vi "DecreaseParameterBounds.vi"(8 "delta":dbl=1.0, 10 "Best Fits":dbl[](array[numeric]), 11 "parameter bounds in":T1={"parameter minimum"=[1.0, 0.0, 0.0, 1.0, 1.0, -720.0, 0.0], "parameter maximum"=[255.0, 640.0, 480.0, 80.0, 80.0, 720.0, 128.0]}) -> (3 "parameter bounds out":T1={"parameter minimum"=[1.0, 0.0, 0.0, 1.0, 1.0, -720.0, 0.0], "parameter maximum"=[255.0, 640.0, 480.0, 80.0, 80.0, 720.0, 128.0]})   [LabVIEW 2015]
panel:
  in  "Amplitude min":dbl=1.0
  # "(0) Amplitude\n(1) X-Pos\n(2) Y-Pos\n(3) width A\n(4) Width B\n(5) angle (DEG)\n(6) Offset"
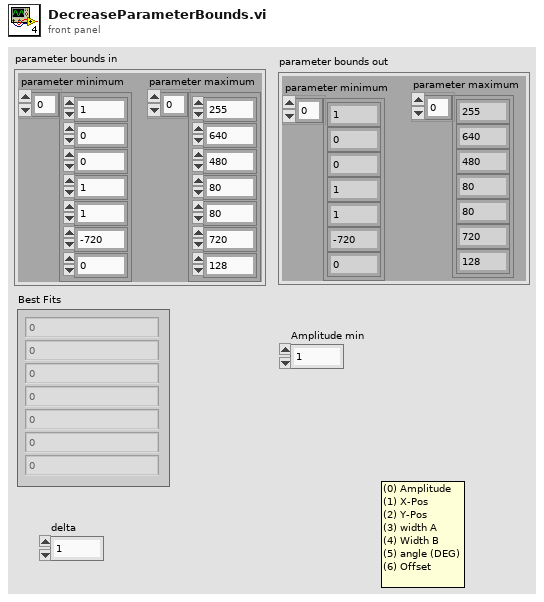
[diagram p1: front panel]
types:
  T1 = cluster{"parameter minimum":dbl[], "parameter maximum":dbl[]}
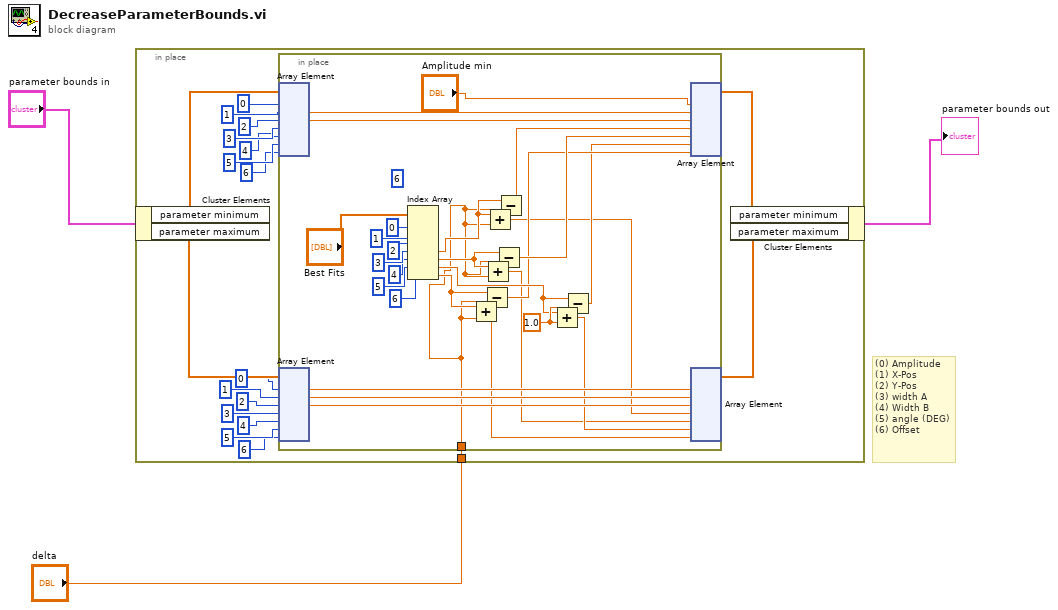
[diagram p0: block diagram]
diagram:
  # "(0) Amplitude\n(1) X-Pos\n(2) Y-Pos\n(3) width A\n(4) Width B\n(5) angle (DEG)\n(6) Offset"
  n1 = in-place {
    in-place-border: "delta" -> [w4]
    n2 = in-place-cluster #1("parameter bounds in") -> ("parameter minimum"=w22:dbl[], "parameter maximum"=w21:dbl[])
    n3 = in-place {
      in-place-border: w4 -> [w23]
      w45 = 1.0 ("y")
      (unwired) 6 ("index")
      n4 = in-place-array #2(w22, 0 ("index"), 1 ("index"), 2 ("index"), 3 ("index"), 4 ("index"), 5 ("index"), 6 ("index")) -> (w47:dbl, w46:dbl)  [unwired: 5 out]
      n5 = in-place-array #3(w21, 0 ("index"), 1 ("index"), 2 ("index"), 3 ("index"), 4 ("index"), 5 ("index"), 6 ("index")) -> (w50:dbl, w49:dbl, w48:dbl)  [unwired: 4 out]
      n6 = Index Array(array="Best Fits", index #1=0 ("index"), index #2=1 ("index"), index #3=2 ("index"), index #4=3 ("index"), index #5=4 ("index"), index #6=5 ("index"), index #7=6 ("index")) -> (element #4=w41:dbl, element #5=w42:dbl, element #6=w44:dbl, element #7=w43:dbl)  [unwired: 3 out]
      n7 = Add(x=w43, y=w23) -> (x+y=w28:dbl)
      n8 = Subtract(x=w43, y=w23) -> (x-y=w31:dbl)
      n9 = Add(x=w42, y=w23) -> (x+y=w26:dbl)
      n10 = Add(x=w41, y=w23) -> (x+y=w29:dbl)
      n11 = Subtract(x=w42, y=w23) -> (x-y=w32:dbl)
      n12 = Subtract(x=w41, y=w23) -> (x-y=w33:dbl)
      n13 = Add(x=w44, y=w45) -> (x+y=w27:dbl)
      n14 = Subtract(x=w44, y=w45) -> (x-y=w30:dbl)
      n15 = in-place-array #2("Amplitude min", w47, w46, w33, w32, w30, w31) -> (w20:dbl[])  [unwired: 7 out]
      n16 = in-place-array #3(w50, w49, w48, w29, w26, w27, w28) -> (w19:dbl[])  [unwired: 7 out]
    }
    n17 = in-place-cluster #1("parameter minimum"=w20, "parameter maximum"=w19) -> (→"parameter bounds out":T1)
  }
